vi "UHR-Fleezers Control (host) - 11.0.vi"() -> ()   [LabVIEW 2011] (continued)
      n2359 = call "downsample 1D array - double.vi"("Ave N"=w3977, "Array In"=w3975) -> ("Array Out"=w3978:dbl[])  [unwired: 1 out]
      n2360 = Bundle By Name(cluster=w3971, "t0"=w3969, "Y"=w3978, "dt"=w3970) -> (w3979:waveform(dbl))
    }
    n2361 = Bundle("BD 1 Frequency 1 (MHz)"=w3195, "BD 1 Frequency 2 (MHz)"=w3194) -> (w3196:T44)  [unwired: 1 out]
    n2362 = call <vilib>:"Mean.vi"("X"=w3229) -> ("mean"=w3217:dbl)  [unwired: 1 out]
    n2363 = call <vilib>:"Mean.vi"("X"=w3230) -> ("mean"=w3218:dbl)  [unwired: 1 out]
    n2364 = Reciprocal(x=w3241) -> (1/x=→"Trap Disp. Freq. (Hz)":dbl)
    n2365 = Cluster To Array(cluster=w3196) -> (array=w3193:dbl[])
    n2366 = local read "Trap X AI1 (DMA)"() -> (w3228:T13)
    n2367 = local read "Data points/scans (MCL)"() -> (w3401:dbl)
    n2368 = To Fixed-Point(number=w3217) -> (fixed-point=w3215:fxp<+/-,16,1>)  [unwired: 1 in]
    n2369 = To Fixed-Point(number=w3218) -> (fixed-point=w3216:fxp<+/-,16,1>)  [unwired: 1 in]
    n2370 = Bundle("Trap 1 Pos.", "Trap 2 Pos.") -> (w3237:cluster{string, string})  [unwired: 1 out]
    n2371 = Bundle By Name(cluster=w3228, "Set 1"=w3216, "Set 2"=w3215) -> (→"Trap X AI1 (DMA)":T13)
    n2372 = Cluster To Array(cluster=w3237) -> (array=w3234:string[])
    n2373 = Bundle("APD 1", "APD 2") -> (w3422:cluster{string, string})  [unwired: 1 out]
    n2374 = Select(t=-1.0, s="Negate Y Axis", f=1.0) -> (s? t:f=w3178:dbl)
    n2375 = for "Trap Position" {
      tunnel: w3243 -> [w3618] mode=indexing
      tunnel: "Trap Pos. Disp. Downsample" -> [w3617]
      tunnel: w3159 -> [w3615]
      tunnel: w3239 -> [w3614]
      tunnel: w3238 -> [w3612]
      tunnel: w3234 -> [w3611] mode=indexing
      tunnel: [w3610] -> w3148 mode=indexing
      tunnel: w3193 -> [w3608] mode=indexing
      tunnel: w3192 -> [w3606]
      tunnel: w3178 -> [w3605]
      n2376 = call "downsample 1D array - double.vi"("Ave N"=w3617, "Array In"=w3618) -> ("Array Out"=w3616:dbl[])  [unwired: 1 out]
      n2377 = Subtract(x=w3616, y=w3608) -> (x-y=w3609:dbl[])
      n2378 = Multiply(x=w3606, y=w3609) -> (x*y=w3607:dbl[])
      n2379 = Multiply(x=w3605, y=w3607) -> (x*y=w3604:dbl[])
      n2380 = Bundle By Name("Y"=w3604, "dt"=w3615, "t0"=w3614) -> (w3613:waveform(dbl))  [unwired: 1 out]
      n2381 = Set Waveform Attribute(5:w3611, 6:w3612, 7:w3613) -> (3:w3610:waveform(dbl))  [unwired: 1 in, 2 out]
    }
    n2382 = Cluster To Array(cluster=w3422) -> (array=w3419:string[])
    n2383 = for "APD" {
      tunnel: w3390 -> [w3958] mode=indexing
      tunnel: w3268 -> [w3966]
      tunnel: [w3962] -> w3275 mode=indexing
      tunnel: "APD Disp. Scale" -> [w3963]
      tunnel: w3238 -> [w3961]
      tunnel: w3419 -> [w3960] mode=indexing
      tunnel: "APD Disp. Downsample" -> [w3956]
      tunnel: [w3959] -> w3418
      workers-P: _ -> [_]
      tunnel: w3239 -> [w3955]
      n2384 = call "integrate 1D array interval - double.vi"("Ave N"=w3956, "Array In"=w3958) -> ("Array Out"=w3957:dbl[])  [unwired: 1 out]
      n2385 = Multiply(x=w3966, y=w3956) -> (x*y=w3959:dbl)
      n2386 = Divide(x=w3957, y=w3963) -> (x/y=w3964:dbl[])
      n2387 = Bundle By Name("t0"=w3955, "Y"=w3964, "dt"=w3959) -> (w3965:waveform(dbl))  [unwired: 1 out]
      n2388 = Set Waveform Attribute(5:w3960, 6:w3961, 7:w3965) -> (3:w3962:waveform(dbl))  [unwired: 1 in, 2 out]
    }
    "APD Display Period (s)" <- w3418
    n2389 = Reciprocal(x=w3418) -> (1/x=→"APD Display Freq. (Hz)":dbl)
    n2390 = local read "Display Period (s)"() -> (w3299:dbl)
    n2391 = Increment(x=w3401) -> (x+1=w3402:dbl)
    n2392 = To Double Precision Float(number=w3311) -> (double precision float=w3310:dbl[])
    n2393 = Index Array(array=w3148, index=0) -> (element=w3152:waveform(dbl))
    n2394 = Index Array(array=w3148, index=1) -> (element=w3147:waveform(dbl))
    n2395 = feedback #7(w3402) -> (w3405:dbl)
    n2396 = Select(t=0, s=w3392, f=w3405) -> (s? t:f=w3398:dbl)
    n2397 = Array Size(array=w3310) -> (size(s)=w3404:i32)
    n2398 = Add(x=w3404, y=w3398) -> (x+y=w3399:dbl)
    n2399 = Unbundle By Name(w3152) -> ("Y"=w3153:dbl[])
    n2400 = feedback #8(w3311) -> (w3388:u32[])
    n2401 = Build Array (concatenate)(w3388, w3311) -> (w3385:u32[])
    n2402 = feedback #9(w3255) -> (w3274:u32[])
    n2403 = Divide(x="Bead Sep. Int. Time (s)", y=w3299) -> (x/y=w3188:dbl)
    n2404 = Build Array (concatenate)(w3274, w3255) -> (w3273:u32[])
    n2405 = Add(x=w3153, y="FB Trap Pos Offset") -> (x+y=w3151:dbl[])
    "T1 x pos data" <- w3151
    n2406 = Greater?(x=w3399, y=w3401) -> (0:w3400:bool)
    n2407 = feedback #10(w3151) -> (w3190:dbl[])
    n2408 = Build Array (concatenate)(w3151, w3190) -> (w3189:dbl[])
    n2409 = Bundle By Name(cluster=w3152, "Y"=w3151) -> (w3150:waveform(dbl))
    n2410 = Select(t=w3398, s=w3400, f=w3399) -> (s? t:f=w3397:dbl)
    n2411 = feedback-in #7(w3397) -> ()
    n2412 = Array Size(array=w3385) -> (size(s)=w3382:i32)
    n2413 = Array Size(array=w3311) -> (size(s)=w3384:i32)
    n2414 = local read "MCL Scanning"() -> (w3395:bool)
    n2415 = local read "APD Integration Time (s)"() -> (w3282:dbl)
    n2416 = Bundle(w3150, w3147) -> (w3146:cluster{waveform(dbl), waveform(dbl)})  [unwired: 1 out]
    n2417 = Build Array (concatenate)(w3275, w3423) -> (w3277:waveform(dbl)[])
    "All Signals" <- w3277
    n2418 = Split 1D Array(array=w3189, index=w3188) -> (first subarray=w3182:dbl[])  [unwired: 1 out]
    n2419 = feedback-in #10(w3182) -> ()
    n2420 = Multiply(x=w3384, y="APD Ave N") -> (x*y=w3383:dbl)
    n2421 = Greater?(x=w3382, y=w3383) -> (0:w3386:bool)
    n2422 = Not(x=w3400) -> (.not. x?=w3394:bool)
    n2423 = Cluster To Array(cluster=w3146) -> (array=→"Trap Positions":waveform(dbl)[])
    n2424 = To Double Precision Float(number=w3255) -> (double precision float=w3254:dbl[])
    n2425 = call <vilib>:"Mean.vi"("X"=w3182) -> ("mean"=w3181:dbl)  [unwired: 1 out]
    "Mean T1 Position (nm)" <- w3181
    n2426 = Subtract(x=w3182, y=w3181) -> (x-y=w3187:dbl[])
    n2427 = Square(x=w3187) -> (x^2=w3186:dbl[])
    n2428 = And(x=w3394, y=w3395) -> (x .and. y?=w3396:bool)
    n2429 = call <vilib>:"Mean.vi"("X"=w3186) -> ("mean"=w3185:dbl)  [unwired: 1 out]
    n2430 = case shown="True" w3386 {
      tunnel: w3385 -> [w3738 w3745]
      tunnel: [w3738 w3743] -> w3328
      tunnel: w3383 -> [_ w3740]
      tunnel: w3382 -> [_ w3744]
      tunnel: w3273 -> [w3737 w3742]
      tunnel: [w3737 w3739] -> w3270
      frame False {
      }
      frame True {
        n2431 = Subtract(x=w3744, y=w3740) -> (x-y=w3741:dbl)
        n2432 = Array Subset(array=w3745, index=w3741, length=w3740) -> (w3743:u32[])
        n2433 = Array Subset(array=w3742, index=w3741, length=w3740) -> (w3739:u32[])
      }
    }
    n2434 = feedback-in #8(w3328) -> ()
    n2435 = feedback-in #9(w3270) -> ()
    n2436 = Square Root(x=w3185) -> (sqrt(x)=w3184:dbl)
    n2437 = Or(x=w3396, y=w3392) -> (x .or. y?=w3393:bool)
    n2438 = Equal?(x="Tab Control 6", y=T34."High Res Display") -> (x = y?=w3317:bool)
    n2439 = Multiply(x="APD Disp. Scale", y=w3275) -> (x*y=w3284:waveform(dbl)[])
    n2440 = Multiply(x=10.0, y=w3184) -> (x*y=→"Trap 1 Position RMS (A)":dbl)
    n2441 = Multiply(x="APD Disp. Downsample", y=w3282) -> (x*y=w3280:dbl)
    n2442 = Divide(x=w3284, y=w3280) -> (x/y=w3252:waveform(dbl)[])
    n2443 = case "For displaying the high resolution display (no downsampling)" shown="True" w3317 {
      tunnel: w3279 -> [_ w3638]
      frame False {
      }
      frame True {
        n2444 = Index Array(array=w3638, index="High Res. Display") -> (element=w3639:waveform(dbl))
        n2445 = call <vilib>:"Std Deviation and Variance.vi"("X"=w3639) -> ("mean"=w3646:dbl, "standard deviation"=w3651:dbl)  [unwired: 1 in, 1 out]
        "Mean Intensity" <- w3646
        "Sigma" <- w3651
        n2446 = Subtract(x=w3639, y=w3646) -> (x-y=w3645:waveform(dbl))
        n2447 = Select(t=w3645, s="Subtract mean", f=w3639) -> (s? t:f=→"1 Channel":waveform(dbl))
        n2448 = Divide(x=w3651, y=w3646) -> (x/y=→"Sigma/Mean":dbl)
        n2449 = feedback #11(1) -> (w3640:i32)
        n2450 = Greater Or Equal?(x=w3640, y="Slow mean N ave.") -> (x >= y?=w3653:bool)
        n2451 = Increment(x=w3640) -> (x+1=w3655:i32)
        n2452 = Select(t=1, s=w3653, f=w3655) -> (s? t:f=w3642:i32)
        n2453 = feedback-in #11(w3642) -> ()
        n2454 = feedback #12() -> (w3643:waveform(dbl))  [unwired: 1 out]
        n2455 = case shown="Default" w3640 {
          tunnel: [w3658 w3661] -> w3644
          tunnel: w3643 -> [w3660 _]
          tunnel: w3639 -> [w3659 w3661]
          frame Default {
            n2456 = call-poly <vilib>:"Append Waveforms.vi"("waveform B"=w3659, "waveform A"=w3660) -> ("waveform out"=w3658:waveform(dbl))  [unwired: 1 in, 8 out]
          }
          frame 1 {
          }
        }
        n2457 = feedback-in #12(w3644) -> ()
        n2458 = case shown="True" w3653 {
          tunnel: w3644 -> [_ w3657]
          frame False {
          }
          frame True {
            n2459 = call <vilib>:"Mean.vi"("X"=w3657) -> ("mean"=→"Slow mean":dbl)  [unwired: 1 out]
          }
        }
      }
    }
    n2460 = Index Array(array=w3252, index=0) -> (element=w3262:waveform(dbl))
    n2461 = Index Array(array=w3252, index=1) -> (element=w3260:waveform(dbl))
    n2462 = case "For computing FFTs for display" shown="True" "Compute FFT" {
      tunnel: w3279 -> [_ w4352]
      frame False {
      }
      frame True {
        n2463 = Build Array("FFT 1 Choice 1", "FFT 1 Choice 2", "FFT 2 Choice 1", "FFT 2 Choice 2") -> (w4345:u16[])
        n2464 = Array Size(array=w4352) -> (size(s)=w4351:i32)
        n2465 = feedback-in #13(w4345) -> ()
        n2466 = feedback #13(u16[] [100, 100, 100, 100]) -> (w4346:u16[])
        n2467 = feedback-in #14("# Spectra to Ave.") -> ()
        n2468 = feedback #14("# Spectra to Ave.") -> (w4343:dbl)
        n2469 = Not Equal?(x="# Spectra to Ave.", y=w4343) -> (x != y?=w4342:bool)
        n2470 = Not Equal?(x=w4345, y=w4346) -> (x != y?=w4344:bool)
        n2471 = feedback #15(1.0) -> (w4329:dbl)
        n2472 = Compound Arithmetic op=OR("Reset FFT", w4344, w4342) -> (w4327:bool)
        n2473 = Select(t=1.0, s=w4327, f=w4329) -> (s? t:f=w4331:dbl)
        n2474 = Greater?(x=w4331, y="# Spectra to Ave.") -> (0:w4350:bool)
        n2475 = Increment(x=w4331) -> (x+1=w4330:dbl)
        n2476 = feedback-in #15(w4330) -> ()
        n2477 = local read "DMA Update Period (s)"() -> (w4325:dbl)
        n2478 = Multiply(x="# Spectra to Ave.", y=w4325) -> (x*y=→"Ave. Time (s)":dbl)
        n2479 = Build Array(cluster{"f0":dbl, "df":dbl, "magnitude":dbl[]} {"f0"=0.0, "df"=0.0, "magnitude"=[]} ("PSD")) -> (w4334:cluster{"f0":dbl, "df":dbl, "magnitude":dbl[]}[])
        n2480 = Build Array(w4334, w4334, w4334, w4334) -> (w4336:T45)
        n2481 = feedback #16(w4336) -> (w4341:T45)
        n2482 = for {
          N: 4 -> [_]
          tunnel: w4345 -> [w4374] mode=indexing
          tunnel: w4352 -> [w4375]
          tunnel: w4351 -> [w4377]
          tunnel: w4327 -> [w4370]
          tunnel: w4350 -> [w4369]
          tunnel: "# Spectra to Ave." -> [w4368]
          tunnel: [w4367] -> w4340 mode=indexing
          tunnel: w4341 -> [w4372] mode=indexing
          tunnel: [w4371] -> w4328 mode=indexing
          tunnel: w4331 -> [w4366]
          n2483 = Less?(x=w4374, y=w4377) -> (x < y?=w4376:bool)
          n2484 = Index Array(array=w4375, index=w4374) -> (element=w4373:waveform(dbl))
          n2485 = case shown="True" w4376 {
            tunnel: w4373 -> [_ w4394]
            tunnel: w4372 -> [w4379 w4392]
            tunnel: [w4379 w4380] -> w4371
            tunnel: w4370 -> [_ w4391]
            tunnel: w4369 -> [_ w4384]
            tunnel: w4368 -> [_ w4383]
            tunnel: [cluster{"f0":dbl, "df":dbl, "magnitude":dbl[]} {"f0"=0.0, "df"=0.0, "magnitude"=[]} ("PSD") w4385] -> w4367
            tunnel: w4366 -> [_ w4382]
            frame False {
            }
            frame True {
              n2486 = call <vilib>:"Std Deviation and Variance.vi"("X"=w4394) -> ("mean"=w4395:dbl)  [unwired: 1 in, 2 out]
              n2487 = Subtract(x=w4394, y=w4395) -> (x-y=w4393:waveform(dbl))
              n2488 = xnode "Spectral Measurements"("Signals"=w4393) -> ("PSD"=w4387:cluster{"f0":dbl, "df":dbl, "magnitude":dbl[]})  [unwired: 1 in, 1 out]
              n2489 = case shown="False" w4391 {
                tunnel: w4392 -> [w4404 _]
                tunnel: [w4400 w4409] -> w4380
                tunnel: w4387 -> [w4403 w4410]
                tunnel: w4384 -> [w4402 _]
                frame False {
                  n2490 = Build Array (concatenate)(w4404, w4403) -> (w4401:cluster{"f0":dbl, "df":dbl, "magnitude":dbl[]}[])
                  n2491 = case shown="True" w4402 {
                    tunnel: w4401 -> [w4405 w4408]
                    tunnel: [w4405 w4406] -> w4400
                    frame False {
                    }
                    frame True {
                      n2492 = Delete From Array(array=w4408, index=0) -> (array with subset deleted=w4406:cluster{"f0":dbl, "df":dbl, "magnitude":dbl[]}[])  [unwired: 1 in, 1 out]
                    }
                  }
                }
                frame True {
                  n2493 = Build Array(w4410) -> (w4409:cluster{"f0":dbl, "df":dbl, "magnitude":dbl[]}[])
                }
              }
              n2494 = for {
                tunnel: w4380 -> [w4399] mode=indexing
                tunnel: [w4398] -> w4390 mode=indexing
                workers-P: _ -> [_]
                n2495 = Unbundle By Name(w4399) -> ("magnitude"=w4398:dbl[])
              }
              n2496 = Transpose 2D Array(2D array=w4390) -> (transposed array=w4389:dbl[][])
              n2497 = for {
                tunnel: w4389 -> [w4397] mode=indexing
                tunnel: [w4396] -> w4388 mode=indexing
                workers-P: _ -> [_]
                n2498 = Add Array Elements(numeric array=w4397) -> (sum=w4396:dbl)
              }
              n2499 = Select(t=w4383, s=w4384, f=w4382) -> (s? t:f=w4381:dbl)
              n2500 = Divide(x=w4388, y=w4381) -> (x/y=w4386:dbl[])
              n2501 = Bundle By Name(cluster=w4387, "magnitude"=w4386) -> (w4385:cluster{"f0":dbl, "df":dbl, "magnitude":dbl[]})
            }
          }
        }
        n2502 = case shown="True" w4327 {
          tunnel: w4328 -> [w4359 w4365]
          tunnel: [w4359 w4360] -> w4326
          frame False {
          }
          frame True {
            n2503 = Array Subset(array=w4365, index (row)=0 ("index"), length (row)=4 ("length"), index (col)=0 ("index"), length (col)=1 ("length")) -> (w4360:T45)
          }
        }
        n2504 = feedback-in #16(w4326) -> ()
        n2505 = Split 1D Array(array=w4340, index=2) -> (first subarray=→"FFT 1":cluster{"f0":dbl, "df":dbl, "magnitude":dbl[]}[], second subarray=→"FFT 2":cluster{"f0":dbl, "df":dbl, "magnitude":dbl[]}[])
      }
    }
    n2506 = case "For plotting results of scanning MCL" shown="True" w3393 {
      tunnel: w3392 -> [_ w3778]
      tunnel: w3310 -> [_ w3874]
      tunnel: w3401 -> [_ _]
      tunnel: w3279 -> [_ w3848]
      tunnel: w3254 -> [_ w3779]
      tunnel: w3253 -> [_ w3752]
      frame False {
      }
      frame True {
        w3759 = u32 0 items=["Horizontal", "Vertical", "Central", "1st Diagonal", "2nd Diagonal"] ("Type of Symmetry")
        w3787 = u32 0 items=["Horizontal", "Vertical", "Central", "1st Diagonal", "2nd Diagonal"] ("Type of Symmetry")
        w3790 = u32 0 items=["Horizontal", "Vertical", "Central", "1st Diagonal", "2nd Diagonal"] ("Type of Symmetry")
        w3819 = u32 0 items=["Horizontal", "Vertical", "Central", "1st Diagonal", "2nd Diagonal"] ("Type of Symmetry")
        n2507 = Index Array(array=w3848, index=10) -> (element=w3854:waveform(dbl))
        n2508 = Index Array(array=w3848, index=11) -> (element=w3851:waveform(dbl))
        n2509 = local read "Cycles/step (MCL)"() -> (w3804:u64)
        n2510 = Index Array(array=w3848, index="Channel") -> (element=w3850:waveform(dbl))
        n2511 = Unbundle(w3752) -> ("New Image"=w3751:T2, "New Image"=w3750:T2, "New Image"=w3749:T2, "New Image"=w3748:T2)
        n2512 = Unbundle By Name(w3854) -> ("Y"=w3806:dbl[])
        n2513 = Unbundle By Name(w3851) -> ("Y"=w3808:dbl[])
        n2514 = Unbundle By Name(w3850) -> ("Y"=w3813:dbl[])
        n2515 = call "downsample 1D array - double.vi"("Ave N"=w3804, "Array In"=w3806) -> ("Array Out"=w3805:dbl[])  [unwired: 1 out]
        n2516 = call "downsample 1D array - double.vi"("Ave N"=w3804, "Array In"=w3808) -> ("Array Out"=w3807:dbl[])  [unwired: 1 out]
        n2517 = call "downsample 1D array - double.vi"("Ave N"=w3804, "Array In"=w3813) -> ("Array Out"=w3812:dbl[])  [unwired: 1 out]
        n2518 = feedback #17(w3874) -> (w3875:dbl[])
        n2519 = Build Array (concatenate)(w3875, w3874) -> (w3856:dbl[])
        n2520 = feedback #18(w3779) -> (w3781:dbl[])
        n2521 = Build Array (concatenate)(w3781, w3779) -> (w3780:dbl[])
        n2522 = local read "Scan steps (MCL)"() -> (w3761:u64)
        n2523 = Select(t=w3874, s=w3778, f=w3856) -> (s? t:f=w3860:dbl[])
        n2524 = feedback-in #17(w3860) -> ()
        n2525 = Select(t=w3779, s=w3778, f=w3780) -> (s? t:f=w3762:dbl[])
        n2526 = feedback-in #18(w3762) -> ()
        n2527 = local read "Scan lines (y)"() -> (w3747:u64)
        n2528 = local read "N APD Samp/step"() -> (w3763:dbl)
        n2529 = feedback #19(w3805) -> (w3862:dbl[])
        n2530 = Build Array (concatenate)(w3862, w3805) -> (w3853:dbl[])
        n2531 = feedback #20(w3812) -> (w3872:dbl[])
        n2532 = Build Array (concatenate)(w3872, w3812) -> (w3871:dbl[])
        n2533 = feedback #21(w3807) -> (w3864:dbl[])
        n2534 = Build Array (concatenate)(w3864, w3807) -> (w3865:dbl[])
        n2535 = Select(t=w3805, s=w3778, f=w3853) -> (s? t:f=w3809:dbl[])
        n2536 = feedback-in #19(w3809) -> ()
        n2537 = Select(t=w3812, s=w3778, f=w3871) -> (s? t:f=w3811:dbl[])
        n2538 = feedback-in #20(w3811) -> ()
        n2539 = Select(t=w3807, s=w3778, f=w3865) -> (s? t:f=w3810:dbl[])
        n2540 = feedback-in #21(w3810) -> ()
        n2541 = Multiply(x=w3761, y=u64 2) -> (x*y=w3746:u64)
        n2542 = call "integrate 1D array interval - double.vi"("Ave N"=w3763, "Array In"=w3762) -> ("Array Out"=w3774:dbl[])  [unwired: 1 out]
        n2543 = call "integrate 1D array interval - double.vi"("Ave N"=w3763, "Array In"=w3860) -> ("Array Out"=w3859:dbl[])  [unwired: 1 out]
        n2544 = Array Size(array=w3774) -> (size(s)=w3775:i32)
        n2545 = Array Size(array=w3859) -> (size(s)=w3861:i32)
        n2546 = Multiply(x=w3747, y=w3746) -> (x*y=w3777:u64)
        n2547 = Multiply(x=w3747, y=w3746) -> (x*y=w3869:u64)
        n2548 = call <vilib>:"Mean.vi"("X"=w3809) -> ("mean"=w3793:dbl)  [unwired: 1 out]
        n2549 = Subtract(x=w3777, y=w3775) -> (x-y=w3768:u64)
        n2550 = call <vilib>:"Mean.vi"("X"=w3811) -> ("mean"=w3798:dbl)  [unwired: 1 out]
        n2551 = call <vilib>:"Mean.vi"("X"=w3810) -> ("mean"=w3796:dbl)  [unwired: 1 out]
        n2552 = call <vilib>:"Mean.vi"("X"=w3774) -> ("mean"=w3765:dbl)  [unwired: 1 out]
        n2553 = Subtract(x=w3869, y=w3861) -> (x-y=w3803:u64)
        n2554 = call <vilib>:"Mean.vi"("X"=w3859) -> ("mean"=w3800:dbl)  [unwired: 1 out]
        n2555 = Initialize Array(1.0 ("element"), w3768) -> (w3764:dbl[])
        n2556 = Initialize Array(1.0 ("element"), w3803) -> (w3794:dbl[])
        n2557 = Multiply(x=w3764, y=w3765) -> (x*y=w3766:dbl[])
        n2558 = Multiply(x=w3794, y=w3796) -> (x*y=w3797:dbl[])
        n2559 = Multiply(x=w3794, y=w3798) -> (x*y=w3799:dbl[])
        n2560 = Multiply(x=w3794, y=w3793) -> (x*y=w3795:dbl[])
        n2561 = Multiply(x=w3794, y=w3800) -> (x*y=w3801:dbl[])
        n2562 = Build Array (concatenate)(w3809, w3795) -> (w3863:dbl[])
        n2563 = Build Array (concatenate)(w3811, w3799) -> (w3867:dbl[])
        n2564 = Build Array (concatenate)(w3810, w3797) -> (w3866:dbl[])
        n2565 = Build Array (concatenate)(w3774, w3766) -> (w3776:dbl[])
        n2566 = Build Array (concatenate)(w3859, w3801) -> (w3868:dbl[])
        n2567 = Reshape Array(w3863, w3747, w3746) -> (w3829:dbl[][])
        n2568 = Reshape Array(w3776, w3747, w3746) -> (w3772:dbl[][])
        n2569 = Reshape Array(w3867, w3747, w3746) -> (w3821:dbl[][])
        n2570 = Reshape Array(w3866, w3747, w3746) -> (w3836:dbl[][])
        n2571 = Reshape Array(w3868, w3747, w3746) -> (w3846:dbl[][])
        n2572 = Array Subset(array=w3836, index (col)=0 ("index"), length (col)=w3761) -> (w3841:dbl[][])  [unwired: 2 in]
        n2573 = Array Subset(array=w3836, index (col)=w3761) -> (w3839:dbl[][])  [unwired: 3 in]
        n2574 = Array Subset(array=w3821, index (col)=0 ("index"), length (col)=w3761) -> (w3827:dbl[][])  [unwired: 2 in]
        n2575 = Array Subset(array=w3821, index (col)=w3761) -> (w3825:dbl[][])  [unwired: 3 in]
        n2576 = Array Subset(array=w3772, index (col)=0 ("index"), length (col)=w3761) -> (w3771:dbl[][])  [unwired: 2 in]
        n2577 = Array Subset(array=w3772, index (col)=w3761) -> (w3769:dbl[][])  [unwired: 3 in]
        n2578 = Array Subset(array=w3846, index (col)=0 ("index"), length (col)=w3761) -> (w3845:dbl[][])  [unwired: 2 in]
        n2579 = Array Subset(array=w3846, index (col)=w3761) -> (w3843:dbl[][])  [unwired: 3 in]
        n2580 = Array Subset(array=w3829, index (col)=0 ("index"), length (col)=w3761) -> (w3834:dbl[][])  [unwired: 2 in]
        n2581 = Array Subset(array=w3829, index (col)=w3761) -> (w3832:dbl[][])  [unwired: 3 in]
        n2582 = for {
          tunnel: w3841 -> [w3883] mode=indexing
          tunnel: [w3882] -> w3840 mode=indexing
          workers-P: _ -> [_]
          n2583 = Reverse 1D Array(array=w3883) -> (reversed array=w3882:dbl[])
        }
        n2584 = for {
          tunnel: w3827 -> [w3879] mode=indexing
          tunnel: [w3878] -> w3826 mode=indexing
          workers-P: _ -> [_]
          n2585 = Reverse 1D Array(array=w3879) -> (reversed array=w3878:dbl[])
        }
        n2586 = for {
          tunnel: w3771 -> [w3877] mode=indexing
          tunnel: [w3876] -> w3770 mode=indexing
          workers-P: _ -> [_]
          n2587 = Reverse 1D Array(array=w3877) -> (reversed array=w3876:dbl[])
        }
        n2588 = for {
          tunnel: w3845 -> [w3885] mode=indexing
          tunnel: [w3884] -> w3844 mode=indexing
          workers-P: _ -> [_]
          n2589 = Reverse 1D Array(array=w3885) -> (reversed array=w3884:dbl[])
        }
        n2590 = for {
          tunnel: w3834 -> [w3881] mode=indexing
          tunnel: [w3880] -> w3833 mode=indexing
          workers-P: _ -> [_]
          n2591 = Reverse 1D Array(array=w3881) -> (reversed array=w3880:dbl[])
        }
        n2592 = Index Array(array=w3846, index (row)=0) -> (element=→"Waveform Graph":dbl[])  [unwired: 1 in]
        n2593 = Add(x=w3840, y=w3839) -> (x+y=w3838:dbl[][])
        n2594 = Add(x=w3826, y=w3825) -> (x+y=w3824:dbl[][])
        n2595 = Add(x=w3770, y=w3769) -> (x+y=w3754:dbl[][])
        n2596 = Add(x=w3844, y=w3843) -> (x+y=w3818:dbl[][])
        n2597 = Add(x=w3833, y=w3832) -> (x+y=w3831:dbl[][])
        n2598 = Divide(x=w3824, y=2) -> (x/y=w3822:dbl[][])
        n2599 = Divide(x=w3838, y=2) -> (x/y=w3783:dbl[][])
        n2600 = Divide(x=w3831, y=2) -> (x/y=w3785:dbl[][])
        n2601 = To Single Precision Float(number=w3818) -> (single precision float=w3817:sgl[][])
        n2602 = Transpose 2D Array(2D array=w3822) -> (transposed array=→"Data map":dbl[][])
        n2603 = To Single Precision Float(number=w3754) -> (single precision float=w3758:sgl[][])
        n2604 = To Single Precision Float(number=w3783) -> (single precision float=w3789:sgl[][])
        n2605 = To Single Precision Float(number=w3785) -> (single precision float=w3786:sgl[][])
        n2606 = call "IMAQ ArrayToImage"("Image Pixels (Float)"=w3817, "Image"=w3751) -> ("Image Out"=w3820:T2)  [unwired: 8 in, 1 out]
        n2607 = call "IMAQ ArrayToImage"("Image Pixels (Float)"=w3758, "Image"=w3750) -> ("Image Out"=w3760:T2)  [unwired: 8 in, 1 out]
        n2608 = call "IMAQ ArrayToImage"("Image Pixels (Float)"=w3789, "Image"=w3749) -> ("Image Out"=w3791:T2)  [unwired: 8 in, 1 out]
        n2609 = call "IMAQ ArrayToImage"("Image Pixels (Float)"=w3786, "Image"=w3748) -> ("Image Out"=w3788:T2)  [unwired: 8 in, 1 out]
        n2610 = call "IMAQ Symmetry"("Type of Symmetry"=w3819, "Image Src"=w3820) -> ("Image Dst Out"=w3815:T2)  [unwired: 3 in, 1 out]
        n2611 = call "IMAQ Symmetry"("Type of Symmetry"=w3759, "Image Src"=w3760) -> ("Image Dst Out"=w3756:T2)  [unwired: 3 in, 1 out]
        n2612 = call "IMAQ Symmetry"("Type of Symmetry"=w3790, "Image Src"=w3791) -> ("Image Dst Out"=→"Detection Laser X":T2)  [unwired: 3 in, 1 out]
        n2613 = call "IMAQ Symmetry"("Type of Symmetry"=w3787, "Image Src"=w3788) -> ("Image Dst Out"=→"Detection Laser Y":T2)  [unwired: 3 in, 1 out]
        n2614 = call "IMAQ Set Simple Calibration"("Calibration Axis Info"=T35 {"Origin Pixel"={"X"=0.0, "Y"=0.0}, "Angle Relative to Horizontal (deg)"=0.0, "Axis Reference"=0}, "Grid Descriptor"=T36 {"X Step"=0.3, "Y Step"=0.3, "Unit"=enum."Undefined"}, "Image"=w3815) -> ("Calibrated Image"=→"APD 1":T2)  [unwired: 7 in, 1 out]
        n2615 = call "IMAQ Set Simple Calibration"("Calibration Axis Info"=T35 {"Origin Pixel"={"X"=0.0, "Y"=0.0}, "Angle Relative to Horizontal (deg)"=0.0, "Axis Reference"=0}, "Grid Descriptor"=T36 {"X Step"=0.3, "Y Step"=0.3, "Unit"=enum."Undefined"}, "Image"=w3756) -> ("Calibrated Image"=→"APD 2":T2)  [unwired: 7 in, 1 out]
      }
    }
    n2616 = Subtract(x=w3260, y="APD 2 Offset") -> (x-y=w3257:waveform(dbl))
    n2617 = Subtract(x=w3262, y="APD 1 Offset") -> (x-y=w3258:waveform(dbl))
    n2618 = Index Array(array=w3277, index=3) -> (element=w3337:waveform(dbl))
    n2619 = Index Array(array=w3277, index=6) -> (element=w3334:waveform(dbl))
    n2620 = Build Array(w3258, w3257) -> (→"APD Chart":waveform(dbl)[])
    n2621 = Array Size(array=w3328) -> (size(s)=w3381:i32)
    n2622 = call <vilib>:"Std Deviation and Variance.vi"("X"=w3270) -> ("standard deviation"=w3269:dbl)  [unwired: 1 in, 2 out]
    n2623 = Add Array Elements(numeric array=w3270) -> (sum=w3272:u32)
    n2624 = Add Array Elements(numeric array=w3328) -> (sum=w3391:u32)
    n2625 = call <vilib>:"Std Deviation and Variance.vi"("X"=w3328) -> ("standard deviation"=w3327:dbl)  [unwired: 1 in, 2 out]
    n2626 = Divide(x="T1 offset_x (mV)", y=1000.0) -> (x/y=w3338:dbl)
    n2627 = Divide(x=w3269, y=w3268) -> (x/y=w3265:dbl)
    "Rate sigma (Hz) 2" <- w3265
    n2628 = Multiply(x=w3268, y=w3381) -> (x*y=w3271:dbl)
    "Int. Time (s)" <- w3271
    n2629 = Divide(x=w3272, y=w3271) -> (x/y=w3266:dbl)
    "APD 2 Rate (Hz)" <- w3266
    n2630 = Divide(x=w3391, y=w3271) -> (x/y=w3325:dbl)
    "APD 1 Rate (Hz)" <- w3325
    n2631 = Divide(x=w3327, y=w3268) -> (x/y=w3326:dbl)
    "Rate sigma (Hz)" <- w3326
    n2632 = Divide(x=w3265, y=w3266) -> (x/y=→"Sigma/Mean 2":dbl)
    n2633 = Divide(x=w3326, y=w3325) -> (x/y=→"Sigma/Mean":dbl)
    n2634 = feedback-in #22("Calibration") -> ()
    n2635 = feedback #22(u16 1 ("Calibration")) -> (w3358:u16)
    n2636 = Divide(x="T2 offset_x (mV)", y=1000.0) -> (x/y=w3336:dbl)
    n2637 = case shown="0, Default" "Calibration" {
      tunnel: "T1 alpha_x (nm/V)" -> [_ w3714 w3735]
      tunnel: "T1 kappa_x (pN/nm)" -> [_ _ w3725]
      tunnel: "T2 alpha_x (nm/V)" -> [_ w3713 w3733]
      tunnel: "T2 kappa_x (pN/nm)" -> [_ _ w3726]
      tunnel: w3337 -> [w3696 w3711 w3731]
      tunnel: w3334 -> [w3695 w3709 w3729]
      tunnel: [w3696 w3708 w3728] -> w3367
      tunnel: [w3695 w3707 w3727] -> w3366
      tunnel: ["T1 X (V)" ("Label.Text") "T1 X (nm)" ("Label.Text") "T1 X (pN)" ("Label.Text")] -> w3355
      tunnel: ["T2 X (V)" ("Label.Text") "T2 X (nm)" ("Label.Text") "T2 X (pN)" ("Label.Text")] -> w3354
      tunnel: ["Position (V)" ("Label.Text") "Position (nm)" ("Label.Text") "Force (pN)" ("Label.Text")] -> w3356
      tunnel: w3336 -> [_ w3699 w3718]
      tunnel: w3338 -> [_ w3702 w3720]
      tunnel: ["Mean (V)" ("Label.Text") "Mean (nm)" ("Label.Text") "Mean (pN)" ("Label.Text")] -> w3351
      tunnel: ["Difference (V)" ("Label.Text") "Difference (nm)" ("Label.Text") "Difference (pN)" ("Label.Text")] -> w3285
      frame 0, Default {
      }
      frame 1 {
        n2638 = Unbundle By Name(w3711) -> ("Y"=w3715:dbl[])
        n2639 = Unbundle By Name(w3709) -> ("Y"=w3700:dbl[])
        n2640 = Subtract(x=w3715, y=w3702) -> (x-y=w3703:dbl[])
        n2641 = Subtract(x=w3700, y=w3699) -> (x-y=w3701:dbl[])
        n2642 = Multiply(x=w3701, y=w3713) -> (x*y=w3710:dbl[])
        n2643 = Multiply(x=w3714, y=w3703) -> (x*y=w3712:dbl[])
        n2644 = Bundle By Name(cluster=w3709, "Y"=w3710) -> (w3707:waveform(dbl))
        n2645 = Bundle By Name(cluster=w3711, "Y"=w3712) -> (w3708:waveform(dbl))
      }
      frame 2 {
        n2646 = Unbundle By Name(w3731) -> ("Y"=w3736:dbl[])
        n2647 = Unbundle By Name(w3729) -> ("Y"=w3734:dbl[])
        n2648 = Subtract(x=w3734, y=w3718) -> (x-y=w3719:dbl[])
        n2649 = Subtract(x=w3736, y=w3720) -> (x-y=w3721:dbl[])
        n2650 = Compound Arithmetic op=MULTIPLY(w3719, w3733, w3726) -> (w3730:dbl[])
        n2651 = Compound Arithmetic op=MULTIPLY(w3725, w3735, w3721) -> (w3732:dbl[])
        n2652 = Bundle By Name(cluster=w3729, "Y"=w3730) -> (w3727:waveform(dbl))
        n2653 = Bundle By Name(cluster=w3731, "Y"=w3732) -> (w3728:waveform(dbl))
      }
    }
    n2654 = Not Equal?(x=w3358, y="Calibration") -> (x != y?=w3315:bool)
    n2655 = case shown="True" w3315 {
      tunnel: w3356 -> [_ w3689]
      tunnel: w3355 -> [_ w3688]
      tunnel: w3354 -> [_ w3687]
      tunnel: w3351 -> [_ w3686]
      tunnel: w3285 -> [_ w3685]
      frame False {
      }
      frame True {
        n2656 = property on="Force" class="WFChart (strict)"("YScale.NameLbl.Text"=w3689) -> ()  [unwired: 2 in, 2 out]
        n2657 = property on="T2 X" class="DigNum (strict)"("Caption.Text"=w3687) -> ()  [unwired: 2 in, 2 out]
        n2658 = property on="T1 X" class="DigNum (strict)"("Caption.Text"=w3688) -> ()  [unwired: 2 in, 2 out]
        n2659 = property on="Mean" class="DigNum (strict)"("Caption.Text"=w3686) -> ()  [unwired: 2 in, 2 out]
        n2660 = property on="Difference" class="DigNum (strict)"("Caption.Text"=w3685) -> ()  [unwired: 2 in, 2 out]
      }
    }
    n2661 = Unbundle By Name(w3337) -> ("Y"=w3340:dbl[])
    n2662 = Unbundle By Name(w3334) -> ("Y"=w3343:dbl[])
    n2663 = Subtract(x=w3340, y=w3338) -> (x-y=w3341:dbl[])
    n2664 = Subtract(x=w3343, y=w3336) -> (x-y=w3342:dbl[])
    n2665 = Multiply(x=w3342, y="T2 alpha_x (nm/V)") -> (x*y=w3126:dbl[])
    n2666 = Multiply(x="T1 alpha_x (nm/V)", y=w3341) -> (x*y=w3127:dbl[])
    n2667 = Not(x="Trap Trig. Fl.") -> (.not. x?=w3164:bool)
    n2668 = Multiply(x=w3366, y=-1.0) -> (x*y=w3345:waveform(dbl))
    n2669 = Subtract(x=w3127, y=w3126) -> (x-y=w3333:dbl[])
    n2670 = Unbundle By Name(w3366) -> ("Y"=w3304:dbl[])
    n2671 = Unbundle By Name(w3367) -> ("Y"=w3128:dbl[])
    n2672 = Negate(x=w3333) -> (-x=w3124:dbl[])
    n2673 = Build Array(w3367, w3345) -> (→"Force":waveform(dbl)[])
    n2674 = Subtract(x=w3124, y="Offset (nm)") -> (x-y=w3302:dbl[])
    n2675 = case shown="True" "Read Lateness and Rel Phase" {
      tunnel: w3144 -> [w3662 w3684]
      tunnel: w3143 -> [w3663 w3683]
      tunnel: [w3662 w3682] -> w3331
      tunnel: [w3663 w3681] -> w3330
      frame False {
      }
      frame True {
        n2676 = xnode "Read/Write Control"("FPGA VI Reference In"=w3684, "error in"=w3683) -> ("FPGA VI Reference Out"=w3682:T19, "error out"=w3681:errorcluster, "GI Relative phase"=→"GI relative phase":i16, "Relative phase"=→"Relative phase (AI1)":i16, "AI Late Counter"=→"Late Counter (AI1)":u16, "GI Late Counter"=→"GI Late Counter":u16, "MCL Late Counter"=→"MCL Late Counter":u16, "MCL Relative Phase"=→"Relative Phase (MCL)":i16, "APD Acq Relative Phase"=→"APD Acq Relative Phase":i16, "APD 1 Gate Relative Phase"=→"APD 1 Gate Relative Phase":i16, "APD 2 Gate Relative Phase"=→"APD 2 Gate Relative Phase":i16, "APD Acq Late Counter"=→"APD Acq Late Counter":u16, "APD 1 Gate Late Counter"=→"APD 1 Gate Late Counter":u16, "APD 2 Gate Late Counter"=→"APD 2 Gate Late Counter":u16, "Green FB Relative Phase"=→"Relative phase (Green FB)":i16, "GI Relative phase 2"=→"GI relative phase 2":i16, "GI Late Counter 2"=→"GI Late Counter 2":u16, "Trap Pos FIFO Timeout"=→"Trap Pos FIFO Timeout":u16, "Trap AI FIFO Timeout"=→"Trap AI FIFO Timeout":u16)
      }
    }
    n2677 = call <vilib>:"Mean.vi"("X"=w3304) -> ("mean"=w3130:dbl)  [unwired: 1 out]
    "T2 X" <- w3130
    n2678 = Negate(x=w3304) -> (-x=w3305:dbl[])
    n2679 = call <vilib>:"Mean.vi"("X"=w3128) -> ("mean"=w3131:dbl)  [unwired: 1 out]
    "T1 X" <- w3131
    n2680 = Negate(x=w3130) -> (-x=w3129:dbl)
    n2681 = Bundle By Name(cluster=w3337, "Y"=w3302) -> (w3276:waveform(dbl))
    "Bead Separation" <- w3276
    n2682 = Add(x=w3128, y=w3305) -> (x+y=w3306:dbl[])
    n2683 = Add(x=w3131, y=w3129) -> (x+y=w3353:dbl)
    n2684 = Subtract(x=w3131, y=w3129) -> (x-y=→"Difference":dbl)
    n2685 = Divide(x=w3306, y=2.0) -> (x/y=→"Vec Mean of T1 T2":dbl[])
    n2686 = Divide(x=w3353, y=2.0) -> (x/y=w3308:dbl)
    "Mean" <- w3308
    n2687 = feedback-in #23("Trap Trig. Fl.") -> ()
    n2688 = feedback #23("Trap Trig. Fl.") -> (w3162:bool)
    n2689 = And(x=w3164, y=w3162) -> (x .and. y?=w3163:bool)
    n2690 = case "If have just turned off triggering" shown="True" w3163 {
      tunnel: w3144 -> [_ w3497]
      tunnel: w3143 -> [_ w3496]
      frame False {
      }
      frame True {
        w3495 = FALSE ("FPGA Trap Trig")
        n2691 = xnode "Read/Write Control"("FPGA VI Reference In"=w3497, "error in"=w3496, "FPGA Trap Trig"=w3495) -> ("FPGA VI Reference Out"=w3494:T19, "error out"=w3493:errorcluster)
        n2692 = xnode "Read/Write Control"("FPGA VI Reference In"=w3494, "error in"=w3493, "TTrig?"=w3495) -> ()  [unwired: 2 out]
        n2693 = local write "Initializing"(FALSE ("Initializing")) -> ()
        n2694 = local write "Triggered"(FALSE ("Triggered")) -> ()
        n2695 = local write "Waiting"(FALSE ("Waiting")) -> ()
      }
    }
    n2696 = Not(x=w3162) -> (.not. x?=w3175:bool)
    n2697 = And(x="Trap Trig. Fl.", y=w3175) -> (x .and. y?=w3172:bool)
    n2698 = local read "Tether"() -> (w3309:bool)
    n2699 = Or(x=w3172, y="Reinitialize") -> (x .or. y?=w3158:bool)
    n2700 = feedback #24(w3168) -> (w3173:string)
    n2701 = Select(t=w3168, s=w3172, f=w3173) -> (s? t:f=w3167:string)
    n2702 = Select(t=w3168, s="Reinitialize", f=w3167) -> (s? t:f=w3166:string)
    n2703 = feedback #25(0) -> (w3170:i32)
    n2704 = feedback #26(w3302) -> (w3301:dbl[])
    n2705 = Build Array (concatenate)(w3302, w3301) -> (w3125:dbl[])
    n2706 = case "For determining if there is a tether still" shown="True" w3309 {
      tunnel: w3308 -> [_ w3621]
      frame False {
      }
      frame True {
        n2707 = Greater?(x="Lost Tether Alarm Threshold (pN)", y=w3621) -> (0:w3619:bool)
        n2708 = case shown="True" w3619 {
          frame False {
          }
          frame True {
            w3622 = FALSE ("Value (Signaling)")
            n2709 = flat-sequence {
              frame #0 {
                # "stop only if saving"
                n2710 = local read "Saving..."() -> (w3634:bool)
                n2711 = And(x=w3634, y="TA Cancel Save?") -> (x .and. y?=w3633:bool)
                n2712 = local write "Stop Saving"(w3633) -> ()
              }
              frame #1 {
                n2713 = case shown="True" "TA Green Off?" {
                  frame False {
                  }
                  frame True {
                    w3637 = FALSE ("Fl. Triggered...")
                    n2714 = local write "Fl. Triggered..."(w3637) -> ()
                    n2715 = property on="Green Laser ON/Interlacing" class="Bool (strict)"("Val(Sgnl)"=w3637) -> ()  [unwired: 2 in, 2 out]
                  }
                }
              }
            }
            n2716 = local read "Time tether formed"() -> (w3628:timestamp)
            n2717 = Get Date/Time In Seconds() -> (seconds since 1Jan1904=w3629:timestamp)
            n2718 = Subtract(x=w3629, y=w3628) -> (x-y=w3627:dbl)
            n2719 = Number To Decimal String(number=w3627) -> (decimal integer string=w3624:string)  [unwired: 1 out]
            n2720 = local read "Messages"() -> (w3631:string)
            n2721 = call <vilib>:"Beep.vi"() -> ()  [unwired: 3 in, 9 out]
            n2722 = Concatenate Strings("Lost tether (" ("Message to add"), w3624, " s)." ("string")) -> (w3626:string)
            n2723 = local write "Tether"(FALSE ("Tether")) -> ()
            n2724 = call "Update messages.vi"("Message to add"=w3626, "Old message string"=w3631) -> ("New message string"=w3630:string)
            n2725 = local write "Messages"(w3630) -> ()
            n2726 = property on="Fl. Triggered..." class="Bool (strict)"("Val(Sgnl)"=w3622) -> ()  [unwired: 2 in, 2 out]
            n2727 = local write "Dip for Protein"(w3622) -> ()
            n2728 = property on="Trap Pos. FB ON" class="Bool (strict)"("Val(Sgnl)"=w3622) -> ()  [unwired: 2 in, 2 out]
            n2729 = property on="Trap Trig. Fl." class="Bool (strict)"("Val(Sgnl)"=w3622) -> ()  [unwired: 2 in, 2 out]
          }
        }
      }
    }
    n2730 = case "For triggering actions based on the trap position (e.g., turning the excitation laser on if trap under feedback moves so far)" shown="True" "Trap Trig. Fl." {
      tunnel: w3153 -> [_ w3510]
      tunnel: w3166 -> [_ w3509]
      tunnel: ["" ("t") w3508] -> w3174
      tunnel: w3158 -> [_ w3507]
      tunnel: [0 ("t") w3506] -> w3171
      tunnel: w3170 -> [_ w3505]
      tunnel: w3144 -> [_ w3504]
      tunnel: w3143 -> [_ w3503]
      frame False {
      }
      frame True {
        n2731 = case shown="\"Wait for trigger\"" w3509 {
          tunnel: w3510 -> [w3527 _ _ w3575]
          tunnel: [w3524 w3556 "" ("t") w3578] -> w3508
          tunnel: w3507 -> [_ _ _ w3566]
          tunnel: [w3523 w3553 0 ("t") w3567] -> w3506
          tunnel: w3505 -> [_ w3555 _ w3573]
          tunnel: w3504 -> [w3512 w3550 _ w3569]
          tunnel: w3503 -> [w3511 w3549 _ w3568]
          frame "Wait for trigger" {
            n2732 = local read "Trap Trig. (FPGA)"() -> (w3515:bool)
            n2733 = Subtract(x=w3527, y="Mean T1 Position\nto compare (nm)") -> (x-y=w3520:dbl[])
            n2734 = call <vilib>:"Std Deviation and Variance.vi"("X"=w3520) -> ("mean"=→"mean":dbl, "standard deviation"=→"standard\ndeviation":dbl)  [unwired: 1 in, 1 out]
            n2735 = Array Max & Min(array=w3520) -> (max value=→"max value":dbl, min value=→"min value":dbl)  [unwired: 2 out]
            n2736 = Greater?(x=w3520, y="Threshold (nm)") -> (0:w3530:bool[])
            n2737 = case shown="True" w3515 {
              tunnel: w3512 -> [_ w3536]
              tunnel: w3511 -> [_ w3535]
              tunnel: [FALSE ("TTrig?") w3534] -> w3518
              frame False {
              }
              frame True {
                n2738 = xnode "Read/Write Control"("FPGA VI Reference In"=w3536, "error in"=w3535) -> ("TTrig?"=w3534:bool)  [unwired: 2 out]
              }
            }
            n2739 = Or Array Elements(Boolean array=w3530) -> (logical OR=w3517:bool)
            n2740 = Select(t=w3518, s=w3515, f=w3517) -> (s? t:f=w3516:bool)
            n2741 = Not(x=w3515) -> (.not. x?=w3514:bool)
            n2742 = And(x=w3516, y=w3514) -> (x .and. y?=w3513:bool)
            n2743 = Select(t="Triggered", s=w3516, f="Wait for trigger") -> (s? t:f=w3524:string)
            n2744 = case shown="True" w3516 {
              tunnel: [0 0] -> w3523
              tunnel: w3512 -> [_ w3541]
              tunnel: w3511 -> [_ w3540]
              frame False {
                "Waiting" <- TRUE ("Waiting")
              }
              frame True {
                n2745 = xnode "Read/Write Control"("FPGA VI Reference In"=w3541, "error in"=w3540, "TTrig?"=FALSE) -> ()  [unwired: 2 out]
                n2746 = local read "Messages"() -> (w3544:string)
                n2747 = call <vilib>:"Beep.vi"() -> ()  [unwired: 12 in]
                n2748 = call "Update messages.vi"("Message to add"="Unwinding trigger.", "Old message string"=w3544) -> ("New message string"=w3545:string)
                n2749 = local write "Messages"(w3545) -> ()
                n2750 = local write "Waiting"(FALSE ("Waiting")) -> ()
                "Triggered" <- TRUE ("Triggered")
              }
            }
            n2751 = case "Only need to turn on laser if host triggered" shown="True" w3513 {
              frame False {
              }
              frame True {
                n2752 = property on="Green Laser ON/Interlacing" class="Bool (strict)"("Val(Sgnl)"=TRUE ("Value (Signaling)")) -> ()  [unwired: 2 in, 2 out]
              }
            }
          }
          frame "Triggered" {
            n2753 = local read "Trap Trig. (FPGA)"() -> (w3552:bool)
            n2754 = Increment(x=w3555) -> (x+1=w3553:i32)
            n2755 = Greater Or Equal?(x=w3553, y="Fl. ON time (n)") -> (x >= y?=w3551:bool)
            n2756 = Select(t="Wait for trigger", s=w3551, f="Triggered" ("t")) -> (s? t:f=w3556:string)
            n2757 = And(x=w3551, y=w3552) -> (x .and. y?=w3548:bool)
            n2758 = case shown="True" w3548 {
              tunnel: w3550 -> [_ w3560]
              tunnel: w3549 -> [_ w3559]
              frame False {
              }
              frame True {
                n2759 = xnode "Read/Write Control"("FPGA VI Reference In"=w3560, "error in"=w3559, "FPGA Trap Trig"=TRUE) -> ()  [unwired: 2 out]
              }
            }
            n2760 = case shown="True" w3551 {
              frame False {
              }
              frame True {
                w3562 = FALSE ("Value (Signaling)")
                n2761 = local write "Triggered"(w3562) -> ()
                n2762 = local write "Waiting"(TRUE ("Waiting")) -> ()
                n2763 = property on="Green Laser ON/Interlacing" class="Bool (strict)"("Val(Sgnl)"=w3562) -> ()  [unwired: 2 in, 2 out]
              }
            }
          }
          frame "Do nothing" {
          }
          frame "Initialize", Default {
            n2764 = Increment(x=w3573) -> (x+1=w3577:i32)
            n2765 = Select(t=1, s=w3566, f=w3577) -> (s? t:f=w3567:i32)
            n2766 = feedback #27(w3575) -> (w3581:dbl[])
            n2767 = Build Array (concatenate)(w3575, w3581) -> (w3574:dbl[])
            n2768 = Greater Or Equal?(x=w3567, y="Wait to get offset (n)") -> (x >= y?=w3570:bool)
            n2769 = Select(t=w3575, s=w3566, f=w3574) -> (s? t:f=w3576:dbl[])
            n2770 = feedback-in #27(w3576) -> ()
            n2771 = call <vilib>:"Mean.vi"("X"=w3576) -> ("mean"=w3571:dbl)  [unwired: 1 out]
            n2772 = local write "Mean T1 Position\nto compare (nm)"(w3571) -> ()
            n2773 = case shown="True" w3566 {
              tunnel: w3569 -> [_ w3587]
              tunnel: w3568 -> [_ w3586]
              frame False {
              }
              frame True {
                w3583 = FALSE ("FPGA Trap Trig")
                n2774 = xnode "Read/Write Control"("FPGA VI Reference In"=w3587, "error in"=w3586, "FPGA Trap Trig"=w3583) -> ("FPGA VI Reference Out"=w3585:T19, "error out"=w3584:errorcluster)
                n2775 = xnode "Read/Write Control"("FPGA VI Reference In"=w3585, "error in"=w3584, "TTrig?"=w3583) -> ()  [unwired: 2 out]
              }
            }
            n2776 = Select(t="Wait for trigger", s=w3570, f="Initialize") -> (s? t:f=w3578:string)
            n2777 = case shown="True" w3570 {
              tunnel: w3571 -> [_ w3590]
              tunnel: w3569 -> [_ w3599]
              tunnel: w3568 -> [_ w3598]
              frame False {
                n2778 = local write "Waiting"(FALSE ("Waiting")) -> ()
                "Initializing" <- TRUE ("Initializing")
              }
              frame True {
                n2779 = local read "Threshold (nm)"() -> (w3602:dbl)
                n2780 = local read "AOM X Cal (nm/MHz)"() -> (w3601:dbl)
                n2781 = Add(x=w3590, y=w3602) -> (x+y=w3603:dbl)
                n2782 = Divide(x=w3603, y=w3601) -> (x/y=w3600:dbl)
                n2783 = call "IR AOM freq to word.vi"("Frequency In (MHz)"=w3600) -> ("Frequency Word Out (double)"=w3597:dbl)
                n2784 = local write "Initializing"(FALSE ("Initializing")) -> ()
                n2785 = local write "Waiting"(TRUE ("Waiting")) -> ()
                n2786 = To Quad Integer(1:w3597) -> (0:w3596:i64)
                n2787 = xnode "Read/Write Control"("FPGA VI Reference In"=w3599, "error in"=w3598, "FPGA TTrig Thresh"=w3596) -> ("FPGA VI Reference Out"=w3593:T19, "error out"=w3592:errorcluster)
                n2788 = xnode "Read/Write Control"("FPGA VI Reference In"=w3593, "error in"=w3592, "FPGA Trap Trig"=TRUE) -> ()  [unwired: 2 out]
              }
            }
          }
        }
      }
    }
    n2789 = feedback-in #24(w3174) -> ()
    n2790 = feedback-in #25(w3171) -> ()
    n2791 = Split 1D Array(array=w3125, index=w3188) -> (first subarray=w3298:dbl[])  [unwired: 1 out]
    n2792 = feedback-in #26(w3298) -> ()
    n2793 = call <vilib>:"Mean.vi"("X"=w3298) -> ("mean"=w3297:dbl)  [unwired: 1 out]
    "Bead Mean (nm)" <- w3297
    n2794 = Subtract(x=w3298, y=w3297) -> (x-y=w3296:dbl[])
    n2795 = Square(x=w3296) -> (x^2=w3295:dbl[])
    n2796 = call <vilib>:"Mean.vi"("X"=w3295) -> ("mean"=w3294:dbl)  [unwired: 1 out]
    n2797 = Square Root(x=w3294) -> (sqrt(x)=w3293:dbl)
    n2798 = Multiply(x=10.0, y=w3293) -> (x*y=→"RMS (Ang)":dbl)
    n2799 = xnode "Read/Write Control"("FPGA VI Reference In"=w3331, "error in"=w3330) -> ("FPGA VI Reference Out"=w3156:T19, "error out"=w3155:errorcluster, "AI2 Y Sum Set 1"=w3437:i16, "AI2 Y Sum Set 2"=w3436:i16, "AI1 X Set 1"=w3220:fxp<+/-,16,1>, "AI1 X Set 2"=w3219:fxp<+/-,16,1>, "Trap Pos FB Int Signal"=→"Trap Pos FB Int Signal":fxp<+/-,24,9>, "Trap Pos FB Int-Norm Signal"=→"Trap Pos FB Int-Norm Signal":fxp<+/-,16,1>, "Trap Pos FB Action"=w3213:i64, "Scanning"=→"AOD Scanning":bool, "Scan I"=→"AOD Scan I":u64, "Scanning MCL"=w3439:bool, "Scan I (MCL)"=→"MCL Scan I":u64, "Green FB Signals"=w3376:T46, "TTrig Sig"=w3142:i64, "TTrig Fin Thresh"=w3138:i64)
    "MCL Scanning" <- w3439
    "Trap Pos FB Action" <- w3213
    n2800 = local read "FB Trig Integrate"() -> (w3136:u32)
    n2801 = Divide(x=w3142, y=w3136) -> (x/y=w3135:dbl)
    "TTrig Sig (Int)" <- w3135
    n2802 = Divide(x=w3138, y=w3136) -> (x/y=w3133:dbl)
    "TTrig Fin Thresh (Int)" <- w3133
    n2803 = local read "AOM X Cal (nm/MHz)"() -> (w3141:dbl)
    n2804 = local read "AI2 (V)"() -> (w3438:cluster{"Set 1":dbl, "Set 2":dbl})
    n2805 = Bundle By Name(cluster=w3438, "Set 1"=w3437, "Set 2"=w3436) -> (w3434:cluster{"Set 1":dbl, "Set 2":dbl})
    n2806 = Divide(x=w3213, y=327.67) -> (x/y=→"Action (%)":dbl)
    n2807 = local read "Trap X (AI1)"() -> (w3233:T10)
    n2808 = call "IR AOM word double to freq.vi"("Frequency Word In (double)"=w3133) -> ("Frequency Out (MHz)"=w3132:dbl)
    n2809 = call "IR AOM word double to freq.vi"("Frequency Word In (double)"=w3135) -> ("Frequency Out (MHz)"=w3134:dbl)
    n2810 = Divide(x=w3434, y=3276.7) -> (x/y=w3433:cluster{"Set 1":dbl, "Set 2":dbl})
    n2811 = Multiply(x=w3134, y=w3141) -> (x*y=w3140:dbl)
    "TTrig Sig (nm)" <- w3140
    n2812 = Multiply(x=w3132, y=w3141) -> (x*y=w3139:dbl)
    "TTrig Fin Thresh (nm)" <- w3139
    n2813 = local write "AI2 (V)"(w3433) -> ()
    n2814 = Bundle(cluster=w3233, "Trap 1"=w3220, "Trap 2"=w3219) -> (→"Trap X (AI1)":T10)
    n2815 = Bundle(w3140, w3139) -> (→"TTrig":cluster{dbl, dbl})  [unwired: 1 in]
    n2816 = Divide(x=w3376, y=3276.7) -> (x/y=w3372:T47)
    n2817 = Unbundle By Name(w3372) -> ("Green FB Ch 0"=w3375:dbl, "Green FB Ch 1"=w3374:dbl, "Green FB Ch 2"=w3373:dbl)
    n2818 = Divide(x=w3375, y=w3373) -> (x/y=w3371:dbl)
    n2819 = Divide(x=w3374, y=w3373) -> (x/y=w3370:dbl)
    n2820 = flat-sequence "To save data" {
      tunnel: [w4458] -> w3457
      tunnel: [w4459] -> w3456
      tunnel: w3407 -> [w4452]
      tunnel: w3161 -> [w4456]
      tunnel: ["Save Calibration"] -> w3430
      tunnel: w3427 -> [w4455]
      tunnel: [w4448] -> w3426
      tunnel: [w4445] -> w3425
      tunnel: [w4442] -> w3424
      tunnel: w3406 -> [w4444]
      tunnel: w3313 -> [w4438]
      tunnel: [w4438] -> w3312
      tunnel: ["Start Saving"] -> w3278
      tunnel: [w4432] -> w3201
      tunnel: [w4431] -> w3200
      tunnel: w3457 -> [w4693]
      tunnel: w3456 -> [w4692]
      tunnel: w3202 -> [w4691]
      tunnel: w3430 -> [w4690]
      tunnel: w3426 -> [w4688]
      tunnel: w3425 -> [w4687]
      tunnel: w3424 -> [w4686]
      tunnel: w3287 -> [w4685]
      tunnel: w3323 -> [w4684]
      tunnel: w3312 -> [w4683]
      tunnel: w3278 -> [w4682]
      tunnel: w3276 -> [w4681]
      tunnel: w3252 -> [w4680]
      tunnel: w3201 -> [w4679]
      tunnel: w3200 -> [w4678]
      tunnel: w3199 -> [w4677]
      frame #0 {
        n2821 = Or(x="Save N Sets", y="Start Saving") -> (x .or. y?=w4439:bool)
        n2822 = To Double Precision Float(number=w4455) -> (double precision float=w4449:dbl)
        n2823 = Build Array(w4439, "Save Calibration", w4452, w4444) -> (w4454:bool[])
        n2824 = Compound Arithmetic op=OR("Save Calibration", w4452, w4439, w4444) -> (w4457:bool)
        n2825 = Boolean Array To Number(Boolean array=w4454) -> (number=w4451:u32)
        n2826 = feedback #28(FALSE ("Save APD Data\nwith Trap Data")) -> (w4433:bool)
        n2827 = feedback #29(refnum<k0> refnum) -> (w4460:refnum<file>)
        n2828 = feedback #30(refnum<k0> refnum) -> (w4435:refnum<file>)
        n2829 = feedback #31(FALSE ("Save APD Data\nwith Trap Data")) -> (w4443:bool)
        n2830 = feedback #32(refnum<k0> refnum) -> (w4446:refnum<file>)
        n2831 = feedback #33(0) -> (w4462:i32)
        n2832 = feedback #34() -> (w4450:u32)  [unwired: 1 out]
        n2833 = case shown="True" w4457 {
          tunnel: [w4469 1] -> w4458
          tunnel: w4462 -> [w4471 _]
          tunnel: [w4470 w4489] -> w4459
          tunnel: w4460 -> [w4470 _]
          tunnel: w4456 -> [_ w4509]
          tunnel: w4449 -> [_ w4507]
          tunnel: w4451 -> [_ w4510]
          tunnel: [w4468 w4488] -> w4448
          tunnel: w4450 -> [w4468 _]
          tunnel: [w4467 w4486] -> w4445
          tunnel: w4446 -> [w4467 _]
          tunnel: [w4466 w4485] -> w4442
          tunnel: w4443 -> [w4466 _]
          tunnel: "Start Saving" -> [_ w4483]
          tunnel: w4438 -> [_ w4482]
          tunnel: [w4465 w4473] -> w4431
          tunnel: w4435 -> [w4465 _]
          tunnel: [w4464 w4472] -> w4432
          tunnel: w4433 -> [w4464 _]
          frame False {
            n2834 = Increment(x=w4471) -> (x+1=w4469:i32)
          }
          frame True {
            w4479 = FALSE ("Start Saving")
            w4484 = 9.0  # File Version
            w4492 = FALSE ("prepend array or string size? (T)")
            w4490 = T24."big-endian, network order" ("byte order (0:big-endian, network order)")
            n2835 = local read "BD 1 Frequency 1 (MHz)"() -> (w4506:dbl)
            n2836 = local read "BD 2 Frequency 1 (MHz)"() -> (w4505:dbl)
            n2837 = local read "BD 1 Frequency 2 (MHz)"() -> (w4504:dbl)
            n2838 = local read "BD 2 Frequency 2 (MHz)"() -> (w4503:dbl)
            n2839 = local read "BD 1 Frequency 3 (MHz)"() -> (w4502:dbl)
            n2840 = local read "BD 2 Frequency 3 (MHz)"() -> (w4501:dbl)
            n2841 = Array Size(array=w4482) -> (size(s)=w4481:i32)
            n2842 = To Double Precision Float(number=w4481) -> (double precision float=w4480:dbl)
            n2843 = local write "Save Calibration"(w4479) -> ()
            n2844 = local write "Start Saving"(w4479) -> ()
            n2845 = Build Array("Save APD Data\nwith Trap Data", "Save Trap Pos. Data") -> (w4476:bool[])
            n2846 = Boolean Array To Number(Boolean array=w4476) -> (number=w4475:u32)
            n2847 = Build Array(w4506, w4505, w4504, w4503, w4502, w4501) -> (w4500:dbl[])
            n2848 = case shown="1, Default" w4510 {
              tunnel: w4509 -> [w4581 w4601 w4617 w4655]
              tunnel: w4480 -> [w4586 w4608 w4637 w4674]
              tunnel: w4507 -> [w4585 w4607 w4636 w4673]
              tunnel: [w4582 w4603 w4628 w4665] -> w4498
              tunnel: [w4573 "Cal sets to save" w4618 w4656] -> w4488
              tunnel: w4500 -> [w4583 w4604 w4630 w4667]
              tunnel: "Save APD Data\nwith Trap Data" -> [w4580 _ w4614 w4653]
              tunnel: [w4580 w4595 w4614 w4653] -> w4485
              tunnel: w4484 -> [w4576 w4596 w4612 w4651]
              tunnel: w4483 -> [w4575 _ _ _]
              tunnel: [w4566 w4595 w4611 w4641] -> w4472
              tunnel: "Save Trap Pos. Data" -> [w4566 _ w4611 w4641]
              tunnel: w4475 -> [w4565 _ w4610 w4640]
              frame 1, Default {
                # "timeseries"
                n2849 = case shown="True" "Profile" {
                  tunnel: [w4589 w4593] -> w4570
                  tunnel: [w4589 w4592] -> w4569
                  tunnel: [w4589 w4591] -> w4568
                  tunnel: [w4589 w4590] -> w4567
                  frame False {
                    w4589 = 0.0 ("f")
                  }
                  frame True {
                    n2850 = local read "Current Position"() -> (w4594:cluster{dbl, dbl, dbl})
                    n2851 = local read "Y change (mm)"() -> (w4590:dbl)
                    n2852 = Unbundle(w4594) -> (w4593:dbl, w4592:dbl, w4591:dbl)
                  }
                }
                n2853 = local read "Save ave N"() -> (w4588:dbl)
                n2854 = Multiply(x=w4588, y=w4581) -> (x*y=w4587:dbl)
                n2855 = To Double Precision Float(number=w4565) -> (double precision float=w4579:dbl)
                n2856 = Build Array(w4576, w4581, w4587, w4586, w4585, 0.0 ("f")) -> (w4584:dbl[])
                n2857 = Build Array(w4579, w4570, w4569, w4568, w4567) -> (w4577:dbl[])
                n2858 = Select(t=u32 4000000000, s=w4575, f="N sets to save") -> (s? t:f=w4573:u32)
                n2859 = Build Array (concatenate)(w4584, w4583, w4577) -> (w4582:dbl[])
              }
              frame 2 {
                w4598 = 0.0 ("f")
                w4595 = FALSE ("Save APD Data\nwith Trap Data")
                # "calibration"
                n2860 = Boolean To (0,1)(Boolean=w4595) -> (0, 1=w4600:i16)
                n2861 = To Double Precision Float(number=w4600) -> (double precision float=w4599:dbl)
                n2862 = Build Array(w4599, w4598, w4598, w4598, w4598) -> (w4597:dbl[])
                n2863 = Build Array(w4596, w4601, w4601, w4608, w4607, 1.0 ("t")) -> (w4605:dbl[])
                n2864 = Build Array (concatenate)(w4605, w4604, w4597) -> (w4603:dbl[])
                "Calibrating Trap..." <- TRUE ("Calibrating...")
              }
              frame 4 {
                w4615 = 0.0 ("f")
                # "scan dir (x/y = 0/1)"
                # "cycles/step"
                # "n scans (f/b)"
                # "steps"
                # "freq. range"
                # "AOD raster scan"
                n2865 = local read "Number of F/B Scans (AOD)"() -> (w4622:u16)
                n2866 = local read "Cycles/step (AOD)"() -> (w4624:u64)
                n2867 = local read "Scan Range (MHz)"() -> (w4627:dbl)
                n2868 = local read "Scan steps (AOD)"() -> (w4626:u64)
                n2869 = local read "Scan BD"() -> (w4634:bool)
                n2870 = local read "Save ave N"() -> (w4639:dbl)
                n2871 = Boolean To (0,1)(Boolean=w4634) -> (0, 1=w4633:i16)
                n2872 = To Double Precision Float(number=w4622) -> (double precision float=w4621:dbl)
                n2873 = To Double Precision Float(number=w4626) -> (double precision float=w4625:dbl)
                n2874 = To Double Precision Float(number=w4624) -> (double precision float=w4623:dbl)
                n2875 = To Double Precision Float(number=w4633) -> (double precision float=w4632:dbl)
                n2876 = Multiply(x=w4639, y=w4617) -> (x*y=w4638:dbl)
                n2877 = To Double Precision Float(number=w4610) -> (double precision float=w4616:dbl)
                n2878 = Build Array(w4616, w4615, w4615, w4615, w4615) -> (w4613:dbl[])
                n2879 = local read "N sets should be saved"() -> (w4619:dbl)
                n2880 = Build Array(w4632, w4627, w4625, w4623, w4621) -> (w4629:dbl[])
                n2881 = Build Array(w4612, w4617, w4638, w4637, w4636, 2.0 ("t")) -> (w4631:dbl[])
                n2882 = Round Toward +Infinity(x=w4619) -> (ceil(x): smallest int >= x=w4620:dbl)
                n2883 = Build Array (concatenate)(w4631, w4630, w4613, w4629) -> (w4628:dbl[])
                n2884 = To Unsigned Long Integer(number=w4620) -> (unsigned 32bit integer=w4618:u32)
              }
              frame 8 {
                w4648 = 0.0 ("f")
                # "MCL raster scan"
                n2885 = local read "Number of scans (MCL)"() -> (w4643:u64)
                n2886 = local read "Scan lines (y)"() -> (w4642:u64)
                n2887 = local read "2D or 1D Scan"() -> (w4645:bool)
                n2888 = local read "Scan Range (V)\n(of steps)"() -> (w4664:dbl)
                n2889 = local read "Fast Scan Dir"() -> (w4671:bool)
                n2890 = local read "Cycles/step (MCL)"() -> (w4661:u64)
                n2891 = local read "Scan steps (MCL)"() -> (w4663:u64)
                n2892 = Select(t=w4642, s=w4645, f=w4643) -> (s? t:f=w4644:u64)
                n2893 = Boolean To (0,1)(Boolean=w4645) -> (0, 1=w4647:i16)
                n2894 = local read "Save ave N"() -> (w4676:dbl)
                n2895 = local read "Initial X"() -> (w4650:dbl)
                n2896 = local read "Initial Y"() -> (w4649:dbl)
                n2897 = To Double Precision Float(number=w4647) -> (double precision float=w4646:dbl)
                n2898 = Boolean To (0,1)(Boolean=w4671) -> (0, 1=w4670:i16)
                n2899 = To Double Precision Float(number=w4644) -> (double precision float=w4659:dbl)
                n2900 = To Double Precision Float(number=w4663) -> (double precision float=w4662:dbl)
                n2901 = To Double Precision Float(number=w4661) -> (double precision float=w4660:dbl)
                n2902 = To Double Precision Float(number=w4670) -> (double precision float=w4669:dbl)
                n2903 = Multiply(x=w4676, y=w4655) -> (x*y=w4675:dbl)
                n2904 = To Double Precision Float(number=w4640) -> (double precision float=w4654:dbl)
                n2905 = local read "N sets should be saved (MCL)"() -> (w4657:dbl)
                n2906 = Build Array(w4654, w4646, w4648, w4648, w4648) -> (w4652:dbl[])
